vi "GetUndoOption.vi"(5 "error in (no error)":errorcluster) -> (15 "UndoSize":i32, 19 "error out":errorcluster)   [LabVIEW 2020, in "UmlEditor.lvclass"]
uses:
  <resource>/Framework/Providers/Open_GDS/UML/UmlEditor_class/UmlEditor.lvclass
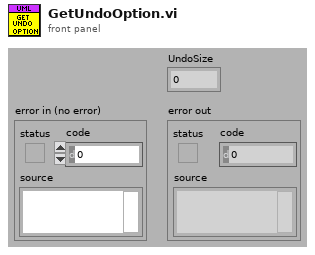
[diagram p1: front panel]
types:
  T1 = typedef "UmlEditor.lvclass/ObjectAttributes.ctl" = cluster{"ListeningQueueIn":refnum<queue>, "Event":refnum<user-event>, "UseProjectFolderAsBasePath":bool, "TypeSyncOption":bool, "Attr":string[], "ToolTip":cluster{"ToolTipOpen":bool, "LastToolTip":i32}, "ClassesToIgnore":string[], "UndoSize":i32, "OpenLastSavedFileWhenStarting":bool, "SyncOption":T2, "SyncTime(s)":i32, "Params":cluster{"IniParams":T3, "Value":string}[], "GraphButtons":refnum<vi>}
  T2 = typedef "UMLEditor_SyncOptions.ctl" = cluster{"IgnoreInstrLib":bool, "IgnoreUserLib":bool, "IgnoreViLib":bool}
  T3 = typedef "UmlEditor.lvclass/IniParamsType.ctl" = enum16{"I have problem with UML stability on my computer"}
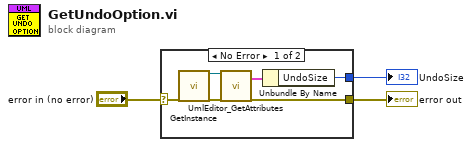
[diagram p0: block diagram]
diagram:
  n1 = case shown="No Error" "error in (no error)" {
    selector: "error in (no error)" -> [w9 w10]
    tunnel: [w6 w10] -> w2
    tunnel: [w5 _] -> w1
    frame No Error {
      n2 = call <resource>:"GetInstance.vi"("error in (no error)"=w9) -> ("reference out"=w8:refnum<class "UmlEditor.lvclass">, "error out"=w7:errorcluster)  [unwired: 17 out]
      n3 = call <resource>:"UmlEditor_GetAttributes.vi"("reference in"=w8, "error in (no error)"=w7) -> ("Data"=w4:T1, "error out"=w6:errorcluster)  [unwired: 1 in, 15 out]
      n4 = Unbundle By Name(w4) -> ("UndoSize"=w5:i32)
    }
    frame Error {
    }
  }
  "error out" <- w2
  "UndoSize" <- w1
